vi "Replace Array Element__ogtk.vi"(7 "New Element":variant, 8 "error in (no error)":errorcluster, 9 "Indices (>=1D)":u32[](array[numeric]), 10 "Index (1D)":u32, 11 "MultiD Array":variant) -> (0 "error out":errorcluster, 2 "VMultiD Array":variant)   [LabVIEW 2016]
doc: "Replaces the elements in a MultiD array at given indices."
panel:
  # "[OpenG VI Tags] ***Do Not Remove***"
  # "Replace Array Element.vi\nPlease visit http://www.OpenG.org to learn about the\nOpen Source LabVIEW software movement.\n\nNOTICE -- YOU MUST LEAVE THIS NOTICE IN PLACE.  PER THE TERMS OF THE LICENSE BELOW, YOU MAY SUBLICENSE THIS SOFTWARE \nIN ANY WAY THAT DOES NOT CONFLICT WITH THIS LICENSE.\n\n### BSD License (http://www.opensource.org/licenses/bsd-license.php) Begin ###\n \nCopyright (c) 2002, Jean-Pierre Drolet <drolet_jp@hotmail.com>\nCopyright (c) 2002-2006, Jim Kring <jim@jimkring.com>\n\nAll rights reserved.\n\nRedistribution and use in source and binary forms, with or without modification, are permitted provided that the following conditions are met:\n\n    * Redistributions of source code must retain the above copyright notice, this list of conditions and the following disclaimer.\n    * Redistributions in binary form must reproduce the above copyright notice, this list of conditions and the following disclaimer in the \n       documentation and/or other materials provided with the distribution.\n    * Neither the name of SciWare, James Kring, Inc., nor the names of its contributors may be used to endorse or promote products derived \n       from this software without specific prior written permission.\n\nTHIS SOFTWARE IS PROVIDED BY THE COPYRIGHT HOLDERS AND CONTRIBUTORS \"AS IS\" AND ANY EXPRESS OR IMPLIED WARRANTIES, \nINCLUDING, BUT NOT LIMITED TO, THE IMPLIED WARRANTIES OF MERCHANTABILITY AND FITNESS FOR A PARTICULAR PURPOSE ARE \nDISCLAIMED. IN NO EVENT SHALL THE COPYRIGHT OWNER OR CONTRIBUTORS BE LIABLE FOR ANY DIRECT, INDIRECT, INCIDENTAL,\n SPECIAL, EXEMPLARY, OR CONSEQUENTIAL DAMAGES (INCLUDING, BUT NOT LIMITED TO, PROCUREMENT OF SUBSTITUTE GOODS OR \nSERVICES; LOSS OF USE, DATA, OR PROFITS; OR BUSINESS INTERRUPTION) HOWEVER CAUSED AND ON ANY THEORY OF LIABILITY, \nWHETHER IN CONTRACT, STRICT LIABILITY, OR TORT (INCLUDING NEGLIGENCE OR OTHERWISE) ARISING IN ANY WAY OUT OF THE USE \nOF THIS SOFTWARE, EVEN IF ADVISED OF THE POSSIBILITY OF SUCH DAMAGE.\n\n### BSD License End ###"
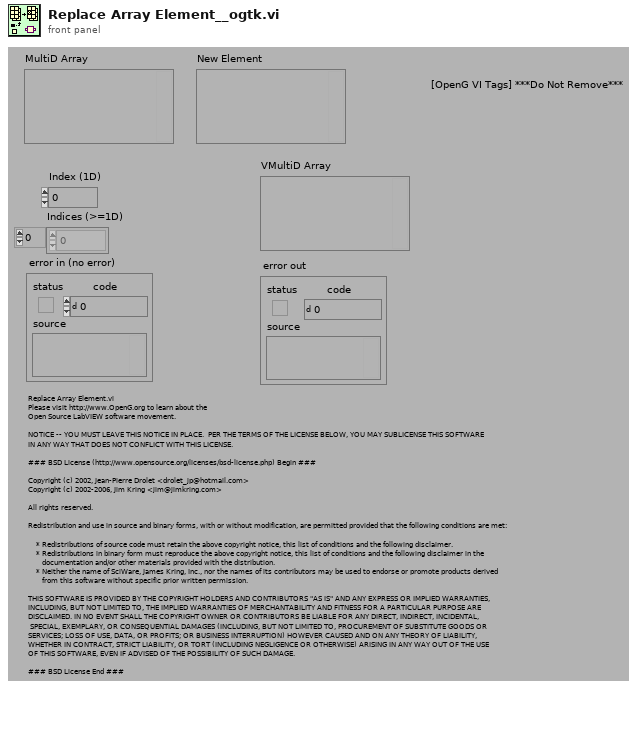
[diagram p1: front panel]
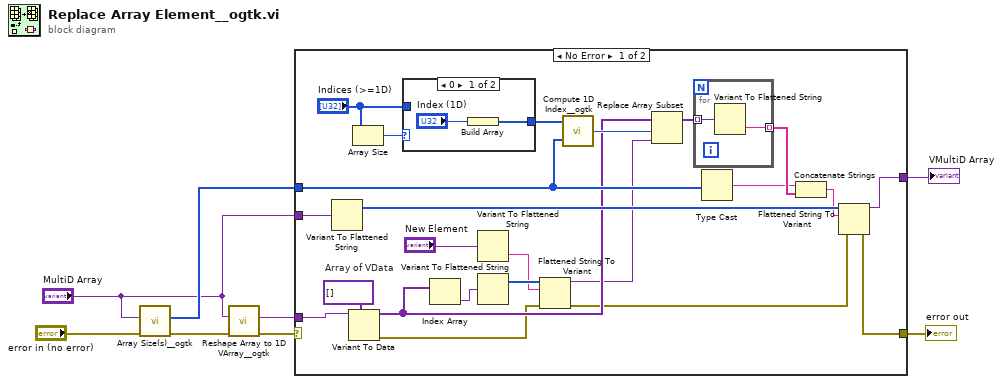
[diagram p0: block diagram]
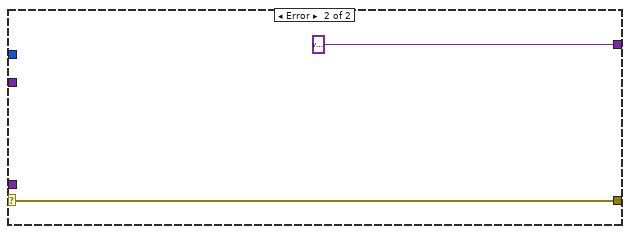
[diagram p3: hidden frame]
diagram:
  n1 = call <userlib>:"Array Size(s)__ogtk.vi"("error in (no error)"="error in (no error)", "Array"="MultiD Array") -> ("error out"=w5:errorcluster, "Size(s)"=w3:u32[])  [unwired: 7 in, 1 out]
  n2 = call <userlib>:"Reshape Array to 1D VArray__ogtk.vi"("error in (no error)"=w5, "MultiD Array"="MultiD Array") -> ("error out"=w7:errorcluster, "1D VArray"=w6:variant)  [unwired: 7 in, 1 out]
  n3 = case shown="No Error" w7 {
    selector: w7 -> [_ w38]
    tunnel: [w19 w38] -> w8
    tunnel: w6 -> [w31 _]
    tunnel: w3 -> [w18 _]
    tunnel: [w20 variant ("MultiD Array")] -> w2
    tunnel: "MultiD Array" -> [w25 _]
    frame No Error {
      w30 = variant[] []  # Array of VData
      n4 = Variant To Flattened String(Variant=w25) -> (1:w22:i16[])  [unwired: 1 out]
      n5 = Variant To Data(type=w30, Variant=w31) -> (data=w16:variant[], error out=w9:errorcluster)  [unwired: 1 in]
      n6 = Array Size(array="Indices (>=1D)") -> (size(s)=w29:i32)
      n7 = case shown="0" w29 {
        tunnel: [w34 w36] -> w27
        tunnel: "Indices (>=1D)" -> [_ w36]
        frame 0 {
          n8 = Build Array("Index (1D)") -> (w34:u32[])
        }
        frame Default {
        }
      }
      n9 = Index Array(array=w16) -> (element=w15:variant)  [unwired: 1 in]
      n10 = Variant To Flattened String(Variant="New Element") -> (data string=w12:string)  [unwired: 1 out]
      n11 = Variant To Flattened String(Variant=w15) -> (1:w13:i16[])  [unwired: 1 out]
      n12 = Flattened String To Variant(4:w9, 6:w12, 7:w13) -> (0:w10:errorcluster, 3:w11:variant)
      n13 = call <userlib>:"Compute 1D Index__ogtk.vi"("Size(s)"=w18, "Indices"=w27) -> ("1D Index"=w26:i32)
      n14 = Replace Array Subset(array=w16, new element=w11, index=w26) -> (w24:variant[])
      n15 = for {
        tunnel: w24 -> [w33] mode=indexing
        tunnel: [w32] -> w23 mode=indexing
        n16 = Variant To Flattened String(Variant=w33) -> (data string=w32:string)  [unwired: 1 out]
      }
      n17 = Type Cast(x=w18) -> (*(type *) &x=w17:string)  [unwired: 1 in]
      n18 = Concatenate Strings(w17, w23) -> (w21:string)
      n19 = Flattened String To Variant(4:w10, 6:w21, 7:w22) -> (0:w19:errorcluster, 3:w20:variant)
    }
    frame Error {
    }
  }
  "error out" <- w8
  "VMultiD Array" <- w2
